vi "LvIRKit_InputIRKitNameAndIP_Panel.vi"(10 "IRKit IP in":string, 11 "IRKit name in":string) -> (1 "Cancel?":bool, 2 "IRKit IP in out":string, 3 "IRKit name out":string)   [LabVIEW 2014]
panel:
  in  "Btn Find":bool
  in  "Btn Cancel":bool
  in  "Btn OK":bool
  in  "IRKit IP":string
  in  "IRKit name":string
  # "IRKitの名前とIPアドレスを入力してください"
  # "IRKitアプリに登録したデバイス名を入力"
  # "nameから検索"
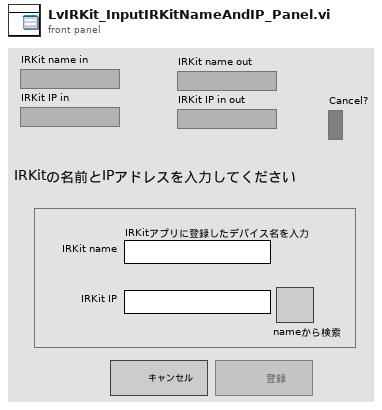
[diagram p1: front panel]
types:
  T1 = enum8{"Enabled", "Disabled", "Disabled and Grayed Out"}
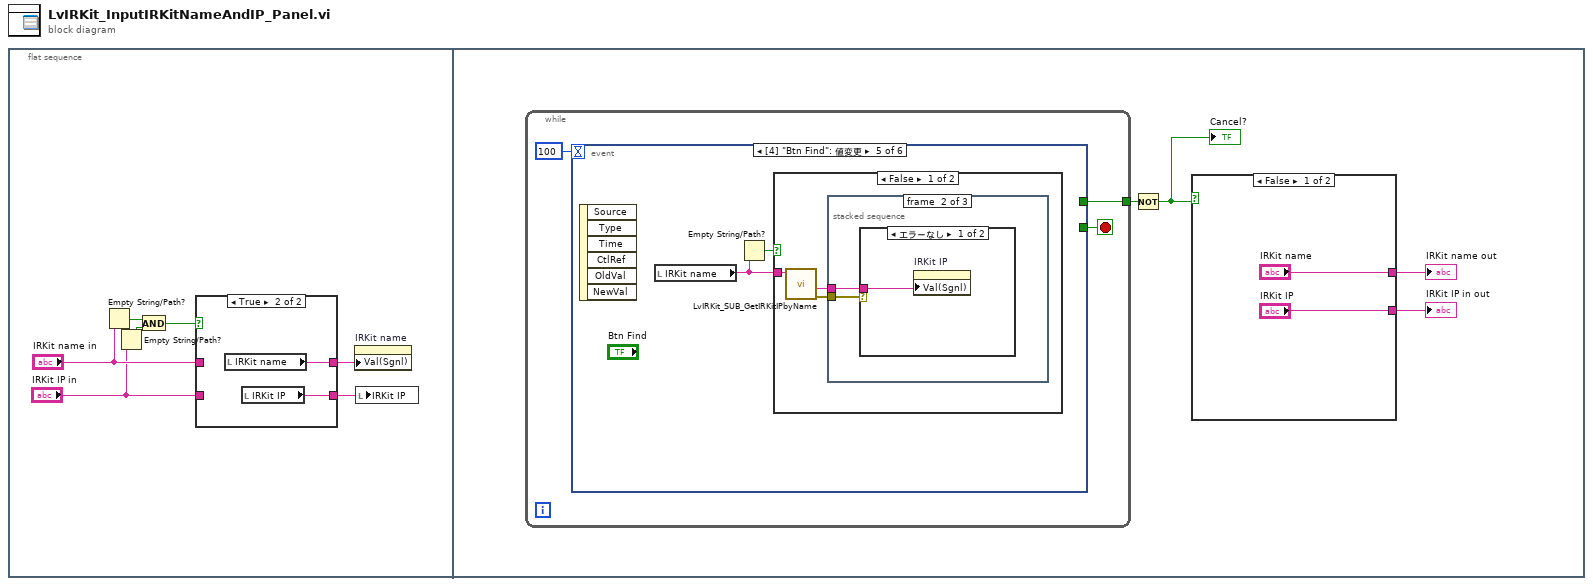
[diagram p0: block diagram]
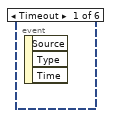
[diagram p4: hidden frame]
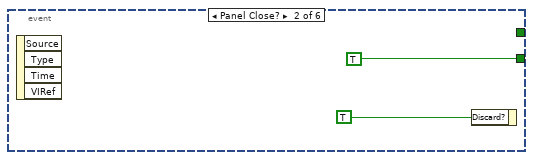
[diagram p5: hidden frame]
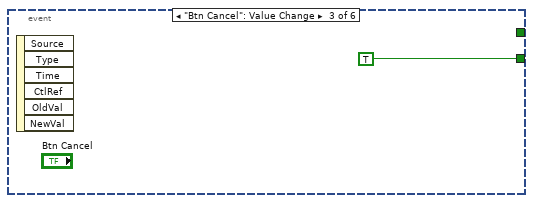
[diagram p6: hidden frame]
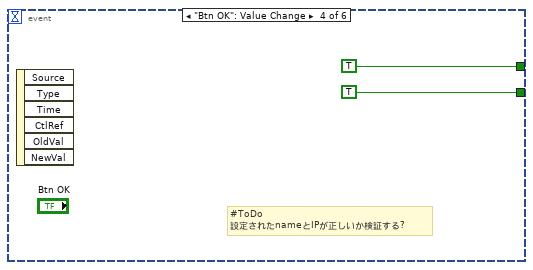
[diagram p7: hidden frame]
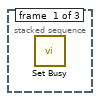
[diagram p8: hidden frame]
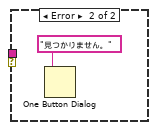
[diagram p9: hidden frame]
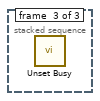
[diagram p10: hidden frame]
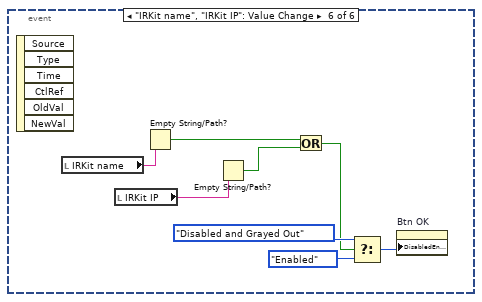
[diagram p12: hidden frame]
diagram:
  n1 = flat-sequence {
    frame #0 {
      n2 = Empty String/Path?(string/path="IRKit name in") -> (empty?=w5:bool)
      n3 = Empty String/Path?(string/path="IRKit IP in") -> (empty?=w1:bool)
      n4 = And(x=w5, y=w1) -> (x .and. y?=w4:bool)
      n5 = case shown="TRUE" w4 {
        tunnel: [w9 w11] -> w7
        tunnel: [w8 w10] -> w6
        tunnel: "IRKit name in" -> [w9 _]
        tunnel: "IRKit IP in" -> [w8 _]
        frame False {
        }
        frame True {
          n6 = local read "IRKit name"() -> (w11:string)
          n7 = local read "IRKit IP"() -> (w10:string)
        }
      }
      n8 = property on="IRKit name" class="Str"("Val(Sgnl)"=w7) -> ()  [unwired: 2 in, 2 out]
      n9 = local write "IRKit IP"(w6) -> ()
    }
    frame #1 {
      n10 = while {
        tunnel: [w18] -> w15
        stop <- w19 stop-if-true
        n11 = event shown="[4] \"Btn Find\": 値変更" {
          selector: _ -> [_ _ _ _ _ _]
          dyn-events: _ -> [_ _ _ _ _ _]
          timeout: 100 -> [_ _ _ _ _ _]
          tunnel: [_ TRUE TRUE TRUE _ _] -> w19
          tunnel: [_ _ _ TRUE _ _] -> w18
          event Timeout {
            n12 = event-data() -> ()  [unwired: 1 in, 3 out]
          }
          event Panel Close? {
            n13 = event-data() -> ()  [unwired: 1 in, 4 out]
            n14 = event-data("Discard?"=TRUE ("破棄?")) -> ()  [unwired: 1 in, 1 out]
          }
          event "Btn Cancel": Value Change {
            n15 = event-data() -> ()  [unwired: 1 in, 6 out]
          }
          event "Btn OK": Value Change {
            # "#ToDo\n設定されたnameとIPが正しいか検証する?"
            n16 = event-data() -> ()  [unwired: 1 in, 6 out]
          }
          event "Btn Find": Value Change {
            n17 = event-data() -> ()  [unwired: 1 in, 6 out]
            n18 = local read "IRKit name"() -> (w27:string)
            n19 = Empty String/Path?(string/path=w27) -> (empty?=w26:bool)
            n20 = case shown="FALSE" w26 {
              tunnel: w27 -> [w30 _]
              frame False {
                n21 = call "LvIRKit_SUB_GetIRKitIPbyName.vi"("IRKit name"=w30) -> ("error out"=w29:errorcluster, "IP"=w28:string)  [unwired: 9 in]
                n22 = stacked-sequence {
                  tunnel: w29 -> [_ w32 _]
                  tunnel: w28 -> [_ w31 _]
                  frame #0 {
                    n23 = call <vilib>:"Set Busy.vi"() -> ()  [unwired: 10 in, 2 out]
                  }
                  frame #1 {
                    n24 = case shown="エラーなし" w32 {
                      tunnel: w31 -> [w33 _]
                      frame No Error {
                        n25 = property on="IRKit IP" class="Str"("Val(Sgnl)"=w33) -> ()  [unwired: 2 in, 2 out]
                      }
                      frame Error {
                        n26 = One Button Dialog(message="見つかりません。" ("メッセージ")) -> ()  [unwired: 1 in, 1 out]
                      }
                    }
                  }
                  frame #2 {
                    n27 = call <vilib>:"Unset Busy.vi"() -> ()  [unwired: 11 in, 1 out]
                  }
                }
              }
              frame True {
              }
            }
          }
          event "IRKit name", "IRKit IP": Value Change {
            n28 = event-data() -> ()  [unwired: 1 in, 6 out]
            n29 = local read "IRKit name"() -> (w36:string)
            n30 = local read "IRKit IP"() -> (w37:string)
            n31 = Empty String/Path?(string/path=w36) -> (empty?=w39:bool)
            n32 = Empty String/Path?(string/path=w37) -> (empty?=w38:bool)
            n33 = Or(x=w39, y=w38) -> (x .or. y?=w35:bool)
            n34 = Select(t=T1."Disabled and Grayed Out" ("無効"), s=w35, f=T1."Enabled" ("無効")) -> (s? t:f=w42:T1)
            n35 = property on="Btn OK" class="Bool"("DisabledEnum"=w42) -> ()  [unwired: 2 in, 2 out]
          }
        }
      }
      n36 = Not(x=w15) -> (.not. x?=w14:bool)
      "Cancel?" <- w14
      n37 = case shown="FALSE" w14 {
        tunnel: ["IRKit name" _] -> w13
        tunnel: ["IRKit IP" _] -> w12
        frame False {
        }
        frame True {
        }
      }
      "IRKit name out" <- w13
      "IRKit IP in out" <- w12
    }
  }
